vi "Start Async.vi"(8 "error in (no error)":errorcluster, 11 "RT Data in":T1 {"Channels"."Voltage"."Ref"."Data Reference" format="%.0x"; "Channels"."Current"."Ref"."Data Reference" format="%.0x"; "Channels"."Read Volt"."Ref" format="%.0x"; "Channels"."Mode"."Ref" format="%.0x"}) -> (0 "error out":errorcluster, 3 "RT Data out":T1 {"Channels"."Voltage"."Ref"."Data Reference" format="%.0x"; "Channels"."Current"."Ref"."Data Reference" format="%.0x"; "Channels"."Read Volt"."Ref" format="%.0x"; "Channels"."Mode"."Ref" format="%.0x"})   [LabVIEW 2011, in "Switch-DMM Custom Device.lvlib"]
uses:
  Switch-DMM Custom Device.lvlib
  Controls/RT Data.ctl
  Controls/Channels.ctl
  Controls/Single Channel.ctl
  <vilib>/NI Veristand/Custom Device API/Data Reference.ctl
  Controls/Block Channels.ctl
  <vilib>/NI Veristand/Custom Device API/Block Data Reference.ctl
  Controls/Communication.ctl
  Controls/Async Status.ctl
  Controls/Async State.ctl
  Controls/Async Command.ctl
  Controls/Async Events.ctl
  <vilib>/NI Veristand/Custom Device API/Custom Device API.lvlib
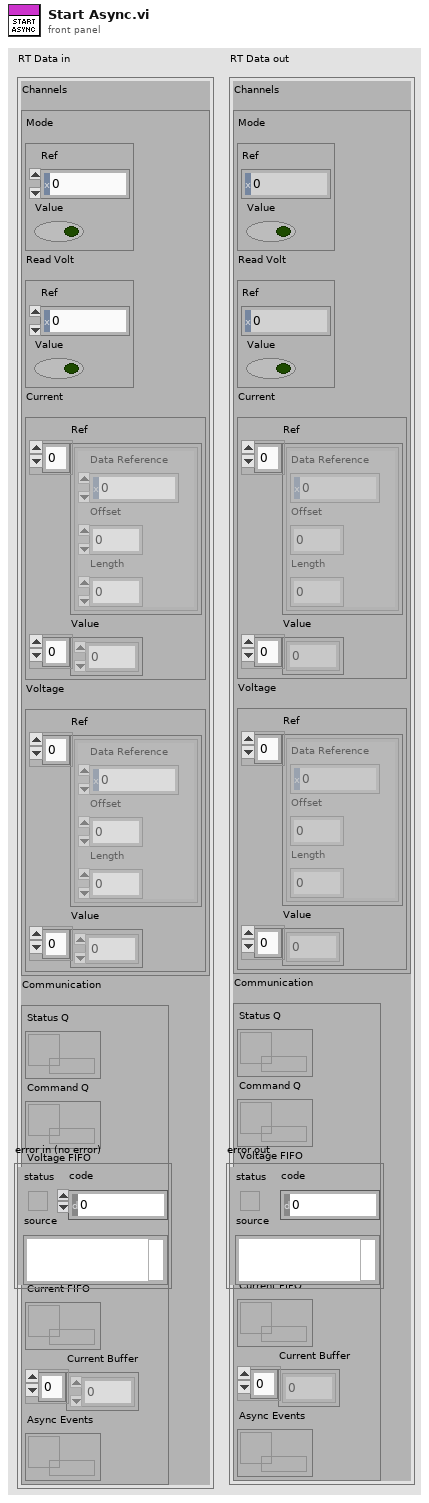
[diagram p1: front panel]
types:
  T1 = typedef "Switch-DMM Custom Device.lvlib/RT Data.ctl" = cluster{"Channels":T2, "Communication":T7}
  T2 = typedef "Switch-DMM Custom Device.lvlib/Channels.ctl" = cluster{"Mode":T3, "Read Volt":T3, "Current":T5, "Voltage":T5}
  T3 = typedef "Switch-DMM Custom Device.lvlib/Single Channel.ctl" = cluster{"Ref":T4, "Value":bool}
  T4 = typedef "Custom Device API.lvlib/Data Reference.ctl" = i32
  T5 = typedef "Switch-DMM Custom Device.lvlib/Block Channels.ctl" = cluster{"Ref":T6[], "Value":dbl[]}
  T6 = typedef "Custom Device API.lvlib/Block Data Reference.ctl" = cluster{"Data Reference":T4, "Offset":i32, "Length":i32}
  T7 = typedef "Switch-DMM Custom Device.lvlib/Communication.ctl" = cluster{"Status Q":refnum<queue>, "Command Q":refnum<queue>, "Voltage FIFO":refnum<k33>, "Voltage Buffer":dbl[], "Current FIFO":refnum<k33>, "Current Buffer":dbl[], "Async Events":refnum<queue>}
  T8 = typedef "Switch-DMM Custom Device.lvlib/Async Command.ctl" = enum16{"None", "Start", "Set Cur Mode", "Req Volt Mode", "Set Volt Mode", "Read Volt", "Exit"}
  T9 = typedef "Switch-DMM Custom Device.lvlib/Async State.ctl" = enum16{"Not running", "Initializing", "Waiting on start cmd", "Running", "Stopped"}
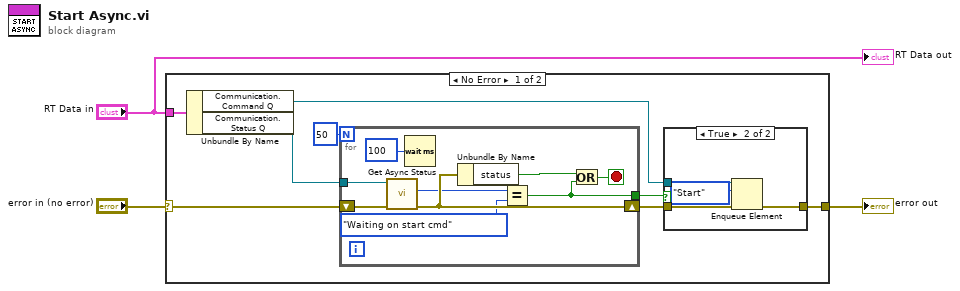
[diagram p0: block diagram]
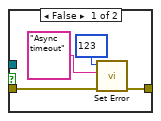
[diagram p2: hidden frame]
diagram:
  n1 = case shown="No Error" "error in (no error)" {
    selector: "error in (no error)" -> [w4 w29]
    tunnel: [w7 w29] -> w3
    tunnel: "RT Data in" -> [w5 _]
    frame No Error {
      n2 = Unbundle By Name(w5) -> ("Communication.Command Q"=w6:refnum<queue>, "Communication.Status Q"=w10:refnum<queue>)
      n3 = for {
        N: 50 -> [_]
        tunnel: w10 -> [w28]
        shift-right: [w25] -> w8
        shift-left: w4 -> [w27]
        tunnel: [w20] -> w9
        stop <- w21 stop-if-true
        n4 = call "Get Async Status.vi"("error in (no error)"=w27, "queue in"=w28) -> ("error out"=w25:errorcluster, "State"=w24:T9)  [unwired: 7 in, 1 out]
        n5 = Wait (ms)(milliseconds to wait=u32 100) -> ()  [unwired: 1 out]
        n6 = Unbundle By Name(w25) -> ("status"=w22:bool)
        n7 = Equal?(x=w24, y=Async_State."Waiting on start cmd" ("State")) -> (x = y?=w20:bool)
        n8 = Or(x=w22, y=w20) -> (x .or. y?=w21:bool)
      }
      n9 = case shown="True" w9 {
        tunnel: w8 -> [w14 w19]
        tunnel: [w12 w18] -> w7
        tunnel: w6 -> [_ w17]
        frame False {
          n10 = call "Set Error.vi"("error in (no error)"=w14, "Message"="Async timeout", "Code"=123) -> ("error out"=w12:errorcluster)  [unwired: 8 in]
        }
        frame True {
          n11 = Enqueue Element(queue=w17, element=Async_Command."Start", error in (no error)=w19) -> (error out=w18:errorcluster)  [unwired: 1 in, 2 out]
        }
      }
    }
    frame Error {
    }
  }
  "error out" <- w3
  "RT Data out" <- "RT Data in"
